vi "GetImage.vi"(0 "XRef":T13, 1 "State In":T3) -> (14 "Image":T2, 15 "Fatal Error Out":T1)   [LabVIEW 2021, in "myRIO AO N Samples Open.xnode"]
uses:
  <vilib>/myRIO/Instrument Drivers/Onboard IO/AO Block/vis/myRIO AO N Samples Open.xnode
  <vilib>/XNodeSupport/XNodeXNodeRef.ctl
  <vilib>/myRIO/Instrument Drivers/Onboard IO/AO Block/vis/State.ctl
  <vilib>/myRIO/Common/Instrument Driver Framework/Utilities/typedefs/myRIOXPeripheral.ctl
  <vilib>/XNodeSupport/XNodeTerm4Array.ctl
  <vilib>/XNodeSupport/XNodeTerm4.ctl
  <vilib>/XNodeSupport/XNodeString.ctl
  <vilib>/XNodeSupport/XNodeVariant.ctl
  <vilib>/XNodeSupport/XNodeRect32.ctl
  <vilib>/XNodeSupport/XNodeInt.ctl
  <vilib>/XNodeSupport/XNodeBool.ctl
  <vilib>/XNodeSupport/XNodeTermDirection.ctl
  <vilib>/XNodeSupport/XNodeImage.ctl
  <vilib>/XNodeSupport/XNodeErrorCluster.ctl
  <vilib>/myRIO/Common/Instrument Driver Framework/Utilities/vis/myRIOXGlobal.vi
  <vilib>/XNodeSupport/NI_XNodeSupport.lvlib
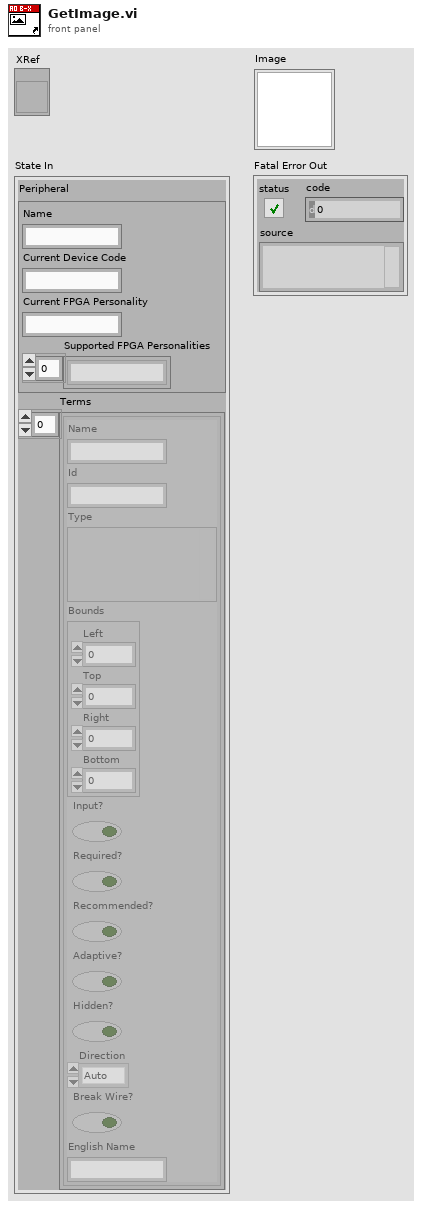
[diagram p1: front panel]
types:
  T1 = typedef "NI_XNodeSupport.lvlib/XNodeErrorCluster.ctl" = errorcluster
  T2 = typedef "NI_XNodeSupport.lvlib/XNodeImage.ctl" = picture
  T3 = typedef "myRIO AO N Samples Open.xnode/State.ctl" = cluster{"Peripheral":T4, "Terms":T5}
  T4 = typedef "myRIOXPeripheral.ctl" = cluster{"Name":string, "Current Device Code":string, "Current FPGA Personality":string, "Supported FPGA Personalities":string[]}
  T5 = typedef "NI_XNodeSupport.lvlib/XNodeTerm4Array.ctl" = T6[]
  T6 = typedef "NI_XNodeSupport.lvlib/XNodeTerm4.ctl" = cluster{"Name":T7, "Id":T7, "Type":T8, "Bounds":T9, "Input?":T11, "Required?":T11, "Recommended?":T11, "Adaptive?":T11, "Hidden?":T11, "Direction":T12, "Break Wire?":T11, "English Name":T7}
  T7 = typedef "NI_XNodeSupport.lvlib/XNodeString.ctl" = string
  T8 = typedef "NI_XNodeSupport.lvlib/XNodeVariant.ctl" = variant
  T9 = typedef "NI_XNodeSupport.lvlib/XNodeRect32.ctl" = cluster{"Left":T10, "Top":T10, "Right":T10, "Bottom":T10}
  T10 = typedef "NI_XNodeSupport.lvlib/XNodeInt.ctl" = i32
  T11 = typedef "NI_XNodeSupport.lvlib/XNodeBool.ctl" = bool
  T12 = typedef "NI_XNodeSupport.lvlib/XNodeTermDirection.ctl" = enum32{"Auto", "Up", "Down", "Left", "Right", "Center"}
  T13 = typedef "NI_XNodeSupport.lvlib/XNodeXNodeRef.ctl" = refnum<vi>
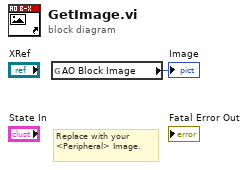
[diagram p0: block diagram]
diagram:
  # "Replace with your <Peripheral> Image."
  n1 = global read "myRIOXGlobal.vi" "AO Block Image"() -> (→"Image":T2)
